vi "Zoom.vi"() -> ()   [LabVIEW 2015]
panel:
  in  "Slider":refnum<vi>
  in  "stop":bool
  in  "ICImagingControl":refnum<k7>(container)
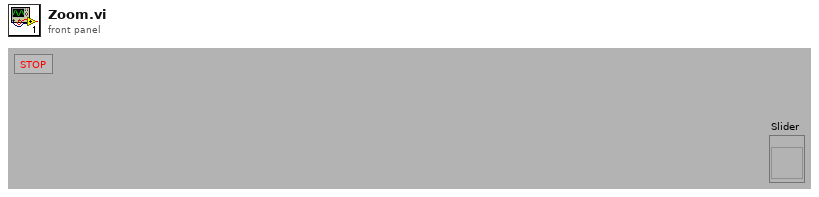
[diagram p1: front panel]
types:
  T1 = enum16{"Brightness", "Color Enable", "Contrast", "Exposure", "Focus", "Gain", "Gamma", "Hue", "Iris", "Pan", "Roll", "Saturation", "Sharpness", "Tilt", "Whitebalance", "Zoom", "Whitebalance Blue", "Whitebalance Red"}
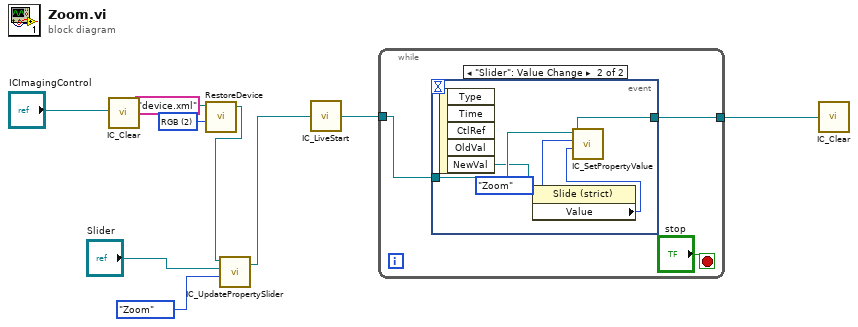
[diagram p0: block diagram]
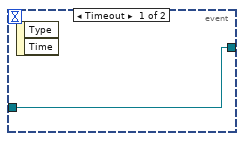
[diagram p2: hidden frame]
diagram:
  w9 = u16 2 items=["RGB"=2, "Y800"=5, "Y16"=11] ("Color modes")
  n1 = call "IC_Clear.vi"("ICImagingControl 2"="ICImagingControl") -> ("ICImagingControl"=w10:refnum<k7>)
  n2 = call "RestoreDevice.vi"("Color modes"=w9, "Filename"="device.xml", "ICImagingControl"=w10) -> ("ICImagingControl 2"=w6:refnum<k7>)  [unwired: 1 in, 2 out]
  n3 = call "IC_UpdatePropertySlider.vi"("Property"=T1."Zoom", "Slider"="Slider", "ICImagingControl In"=w6) -> ("ICImagingControl Out"=w5:refnum<k7>)  [unwired: 1 in, 1 out]
  n4 = call "IC_LiveStart.vi"("ICImagingControl 3"=w5) -> ("ICImagingControl 2"=w7:refnum<k7>)
  n5 = while {
    tunnel: w7 -> [w12]
    tunnel: [w11] -> w2
    stop <- "stop" stop-if-true
    n6 = event shown="[1] \"Slider\": Value Change" {
      selector: _ -> [_ _]
      dyn-events: _ -> [_ _]
      timeout: _ -> [_ _]
      tunnel: w12 -> [w14 w19]
      tunnel: [w14 w18] -> w11
      event Timeout {
        n7 = event-data() -> ()  [unwired: 1 in, 2 out]
      }
      event "Slider": Value Change {
        n8 = event-data() -> ("NewVal"=w16:refnum<vi>)  [unwired: 1 in, 4 out]
        n9 = property class="Slide (strict)"(reference=w16) -> ("Value"=w15:i32)  [unwired: 1 in, 2 out]
        n10 = call "IC_SetPropertyValue.vi"("Value"=w15, "Property"=T1."Zoom", "ICImagingControl In"=w19) -> ("ICImagingControl Out"=w18:refnum<k7>)  [unwired: 1 in, 1 out]
      }
    }
  }
  n11 = call "IC_Clear.vi"("ICImagingControl 2"=w2) -> ()  [unwired: 1 out]
